vi "Inject Command Directors.vi"(8 "error in (no error)":errorcluster, 10 "Injected Command Directors":refnum<class "CommandDirector.lvclass">[](array[class]), 11 "TestProcessor in":refnum<class "TestProcessor.lvclass">) -> (0 "error out":errorcluster, 3 "TestProcessor out":refnum<class "TestProcessor.lvclass">)   [LabVIEW 2023, in "HAF.lvlib" / "TestProcessor.lvclass"]
doc: "Add the passed Command Directors to the Test. These will be added to the end of the existing Command Directors which will continue to run, i.e. nothing is replaced. Note that unless the Test Processor has been told to expect injections, it may finished before this can happen: Handle Injections should be set to True as part of running the test."
uses:
  TestProcessor.lvclass
  TestProcessor.lvclass/TestProcessor.ctl
  HAF.lvlib
  CommandDirector/CommandDirector.lvclass
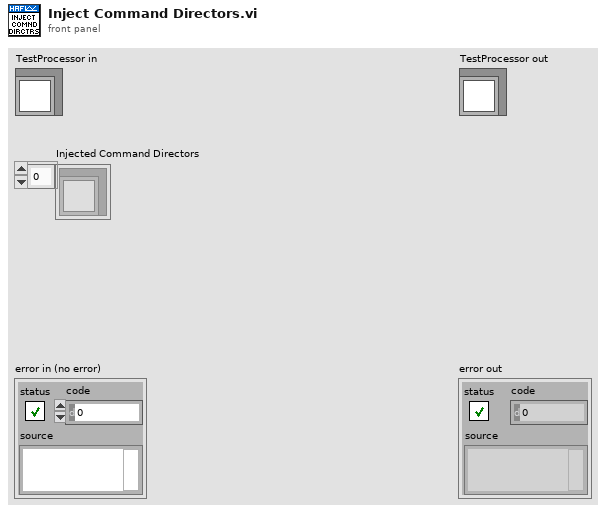
[diagram p1: front panel]
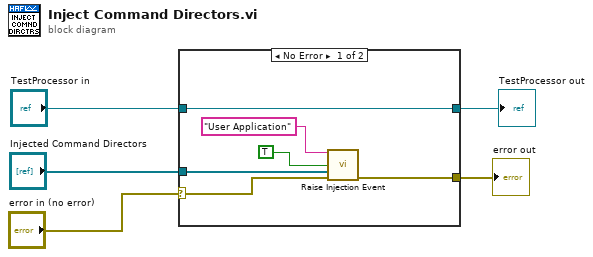
[diagram p0: block diagram]
diagram:
  n1 = case shown="No Error" "error in (no error)" {
    selector: "error in (no error)" -> [w8 w13]
    tunnel: [w7 w13] -> w4
    tunnel: [w11 w12] -> w2
    tunnel: "TestProcessor in" -> [w11 w12]
    tunnel: "Injected Command Directors" -> [w6 _]
    frame No Error {
      n2 = call "Raise Injection Event.vi"("Raiser Name"="User Application", "Send Injection"=TRUE, "Injected Command Directors"=w6, "error in (no error)"=w8) -> ("error out"=w7:errorcluster)  [unwired: 11 in]
    }
    frame Error {
    }
  }
  "error out" <- w4
  "TestProcessor out" <- w2
